vi "Create Line Sized Linear Array.vi"(8 "error in (no error)":errorcluster, 11 "Line Sizes (unreleased)":refnum<class "1D Array f32.lvclass">) -> (0 "error out":errorcluster, 2 "Max Line Size":i32, 3 "Line Sized Linear Array":refnum<class "2D Array f32.lvclass">)   [LabVIEW 2024, in "G2CPU Line Profile.lvlib"]
uses:
  G2CPU Line Profile.lvlib
  <vilib>/Natan Biesmans/G2CPU GPU and CPU HPC Toolkit/G2CPU Libraries/Arrays/2DArray/f32/2D Array f32.lvclass
  C:/Program Files/National Instruments/LabVIEW 2025/vi.lib/Natan Biesmans/G2CPU GPU and CPU HPC Toolkit/G2CPU Libraries/Arrays/Array/Array Prototype.lvclass
  <vilib>/Natan Biesmans/G2CPU GPU and CPU HPC Toolkit/G2CPU Libraries/Arrays/1DArray/f32/1D Array f32.lvclass
  a4cb5a3b-36b7-4582-90a9-cb480767becf.vi
  64dc8cec-d612-45ea-a810-79d2c8018071.vi
  a4cb5a3b-36b7-4582-90a9-cb480767becf.vi/72eb0651-ae32-4ba2-a447-070823507cb2.vi
  64dc8cec-d612-45ea-a810-79d2c8018071.vi/ab6cfe59-c8ad-4da3-839b-8d02ec9e015f.vi
  64dc8cec-d612-45ea-a810-79d2c8018071.vi/ab6cfe59-c8ad-4da3-839b-8d02ec9e015f.vi/313ec8c5-c203-475c-9de0-0583f6fb8b4d.vi
  <vilib>/Natan Biesmans/G2CPU GPU and CPU HPC Toolkit/G2CPU Libraries/Arrays/Array/G2CPU Lock Array.vi
  <vilib>/Natan Biesmans/G2CPU GPU and CPU HPC Toolkit/G2CPU Libraries/Arrays/Array/G2CPU Get Array Pointer.vi
  <vilib>/Natan Biesmans/G2CPU GPU and CPU HPC Toolkit/ArrayFire Driver/VIs/max all.vi
  <vilib>/Natan Biesmans/G2CPU GPU and CPU HPC Toolkit/G2CPU Libraries/Arrays/Array/G2CPU Unlock Array.vi
  <vilib>/Natan Biesmans/G2CPU GPU and CPU HPC Toolkit/G2CPU Libraries/Arrays/Array/G2CPU Release Array.vi
  <vilib>/Natan Biesmans/G2CPU GPU and CPU HPC Toolkit/ArrayFire Driver/VIs/range.vi
  <vilib>/Natan Biesmans/G2CPU GPU and CPU HPC Toolkit/G2CPU Libraries/Arrays/Array/G2CPU Set Array Pointer.vi
  <vilib>/Natan Biesmans/G2CPU GPU and CPU HPC Toolkit/G2CPU Libraries/Arrays/Array/Array Prototype.lvclass
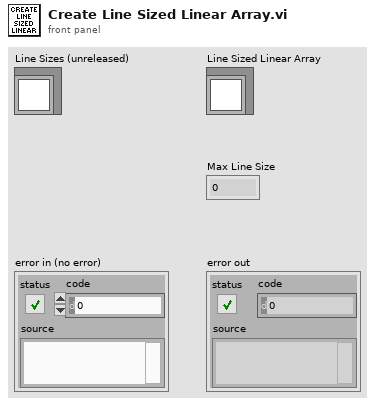
[diagram p1: front panel]
types:
  T1 = typedef "AF.lvlib/Dim4.ctl" = cluster{"Dim 0":u64, "Dim 1":u64, "Dim 2":u64, "Dim 3":u64}
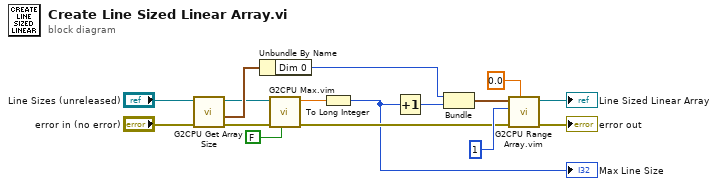
[diagram p0: block diagram]
diagram:
  n1 = call <vilib>:"G2CPU Get Array Size.vi"("error in (no error)"="error in (no error)", "Array in"="Line Sizes (unreleased)") -> ("error out"=w6:errorcluster, "Array Size"=w10:T1, "Array out"=w7:refnum<class "1D Array f32.lvclass">)  [unwired: 6 in, 1 out]
  n2 = Unbundle By Name(w10) -> ("Dim 0"=w11:u64)
  n3 = call "G2CPU Max.vim"("Auto Release (Enabled)"=FALSE, "error in (no error)"=w6, "Array First"=w7) -> ("error out"=w5:errorcluster, "real out"=w15:dbl)  [unwired: 6 in, 1 out]
  n4 = To Long Integer(number=w15) -> (32bit integer=w2:i32)
  "Max Line Size" <- w2
  n5 = Increment(x=w2) -> (x+1=w14:i32)
  n6 = Bundle("Dim 0"=w11, w14) -> (w9:cluster{"Dim 0":u64, i32})  [unwired: 1 in]
  n7 = call "G2CPU Range Array.vim"("Datatype"=sgl 0.0, "Error in"=w5, "Sequential Dimension"=1, "Size"=w9) -> ("error out"=→"error out":errorcluster, "Array out"=→"Line Sized Linear Array":refnum<class "2D Array f32.lvclass">)  [unwired: 6 in]
